vi "Output Character Codes.vi"(8 "error in (no error)":errorcluster, 9 "position":cluster{"row":i8, "column":i8}, 10 "character codes":u8[](array[numeric]), 11 "HD44780 in":refnum<class "HD44780.lvclass">) -> (0 "error out":errorcluster, 1 "current cursor position":cluster{"row":i8, "column":i8}, 3 "HD44780 out":refnum<class "HD44780.lvclass">)   [LabVIEW 2017, in "HD44780.lvclass"]
uses:
  HD44780.lvclass
  HD44780.lvclass/HD44780.ctl
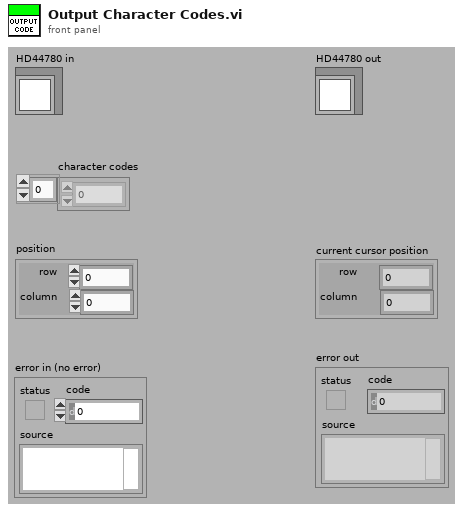
[diagram p1: front panel]
types:
  T1 = typedef "HD44780 Common.lvlib/cluster of class private data.ctl" = cluster{"FPGA VI Reference":refnum<k20>, "device index":i8, "screen size":T2, "font size":T3, "auto wrap":bool, "alignment":T4, "number of line":T5, "shift 0":i8, "entry mode 0":T6, "shift 1":i8, "entry mode 1":T6}
  T2 = typedef "HD44780 Common.lvlib/screen size.ctl" = enum8{"8x1", "8x2", "12x4", "16x1", "16x2", "16x4", "20x1", "20x2", "20x4", "24x1", "24x2", "40x2", "40x4"}
  T3 = typedef "HD44780 Common.lvlib/font size.ctl" = enum8{"5x8", "5x10"}
  T4 = typedef "HD44780 Common.lvlib/alignment.ctl" = enum16{"None", "Left", "Center", "Right"}
  T5 = typedef "HD44780 Common.lvlib/line number.ctl" = enum8{"1 line", "2 lines"}
  T6 = typedef "HD44780 Common.lvlib/entry mode.ctl" = enum8{"increment & no shift", "increment & shift", "decrement & no shift", "decrement & shift"}
  T7 = cluster{"FPGA VI Reference":refnum<k20>, "device index":i8, "screen size":enum8{"8x1", "8x2", "12x4", "16x1", "16x2", "16x4", "20x1", "20x2", "20x4", "24x1", "24x2", "40x2", "40x4"}, "font size":enum8{"5x8", "5x10"}, "auto wrap":bool, "alignment":enum16{"None", "Left", "Center", "Right"}, "number of line":enum8{"1 line", "2 lines"}, "shift 0":i8, "entry mode 0":enum8{"increment & no shift", "increment & shift", "decrement & no shift", "decrement & shift"}, "shift 1":i8, "entry mode 1":enum8{"increment & no shift", "increment & shift", "decrement & no shift", "decrement & shift"}}
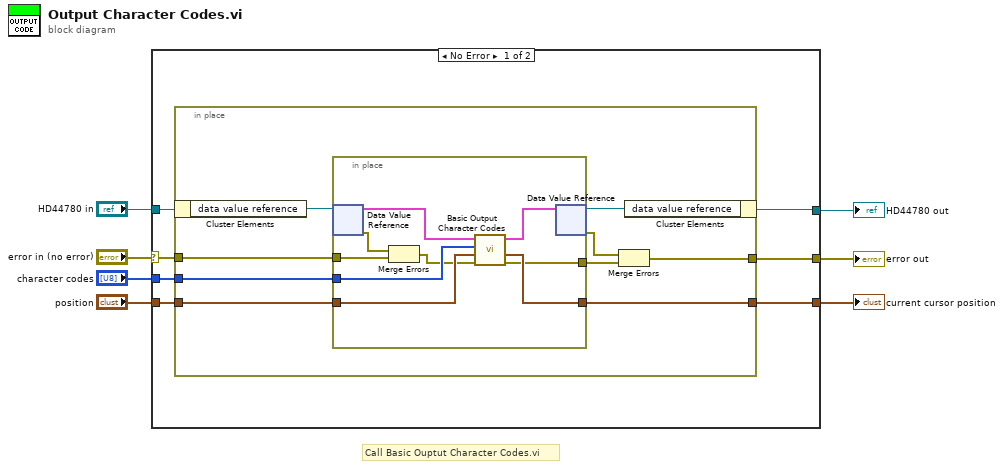
[diagram p0: block diagram]
diagram:
  # "Call Basic Ouptut Character Codes.vi"
  n1 = case shown="No Error" "error in (no error)" {
    selector: "error in (no error)" -> [w8 w35]
    tunnel: [w10 w35] -> w1
    tunnel: "position" -> [w14 w34]
    tunnel: "character codes" -> [w13 _]
    tunnel: "HD44780 in" -> [w11 w33]
    tunnel: [w12 w34] -> w4
    tunnel: [w9 w33] -> w2
    frame No Error {
      n2 = in-place {
        in-place-border: w14 -> [w20]
        in-place-border: w13 -> [w21]
        in-place-border: [w23] -> w12
        in-place-border: [w17] -> w10
        in-place-border: w8 -> [w16]
        n3 = in-place-cluster #1(w11) -> ("data value reference"=w22:refnum<data-value>)
        n4 = in-place {
          in-place-border: [w32] -> w23
          in-place-border: w21 -> [w30]
          in-place-border: w20 -> [w31]
          in-place-border: w16 -> [w28]
          in-place-border: [w26] -> w15
          n5 = in-place-dvr #2(w22) -> (w25:T1, w29:errorcluster)
          n6 = Merge Errors(w29, w28) -> (w24:errorcluster)
          n7 = call "Basic Output Character Codes.vi"("error in (no error)"=w24, "position (0, 0)"=w31, "character codes"=w30, "cluster of class private data in"=w25) -> ("error out"=w26:errorcluster, "current position"=w32:cluster{"row":i8, "column":i8}, "cluster of private data out"=w27:T7)  [unwired: 5 in]
          n8 = in-place-dvr #2(w27) -> (w19:refnum<data-value>, w18:errorcluster)
        }
        n9 = Merge Errors(w18, w15) -> (w17:errorcluster)
        n10 = in-place-cluster #1("data value reference"=w19) -> (w9:refnum<class "HD44780.lvclass">)
      }
    }
    frame Error {
    }
  }
  "error out" <- w1
  "HD44780 out" <- w2
  "current cursor position" <- w4
